vi "New1009.vi"   [LabVIEW 2013]
uses:
  <vilib>/Heliosphere Research LLC/Advanced Plotting Toolkit/api_core/NewPlotScales.ctl
  <vilib>/Heliosphere Research LLC/Advanced Plotting Toolkit/Advanced Plotting Toolkit.lvlib
types:
  T1 = typedef "Advanced Plotting Toolkit.lvlib/NewPlotScales.ctl" = enum16{"Default", "Linear", "Log", "Symlog"}
  T2 = typedef "Advanced Plotting Toolkit.lvlib/PlotID.ctl" = i32
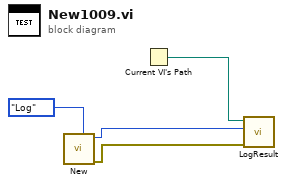
[diagram p0: block diagram]
diagram:
  n1 = call <vilib>:"New.vi"("Y Axis Scale"=NewPlotScales."Log" ("X Axis Scale")) -> ("error out"=w2:errorcluster, "Plot ID"=w3:T2)  [unwired: 9 in]
  n2 = Current VI's Path() -> (path=w4:path)
  n3 = call "LogResult.vi"("Test Result"=w2, "Test Artifact"=w3, "VI Path"=w4) -> ()  [unwired: 9 in]
